vi "Zaxis_ZRaxis_Test.vi"() -> ()   [LabVIEW 2019]
uses:
  WSCbot_V3_Toolkit.lvlibp/WSCBOTV3_Toolkit/MotorControl/LowLevel/ZaxisSlideSet.vi
  WSCbot_V3_Toolkit.lvlibp/WSCBOTV3_Toolkit/MotorControl/LowLevel/ZRaxisRotatingSet.vi
  WSCbot_V3_Toolkit.lvlibp
panel:
  in  "TargetHight(deg)":dbl format="%#_13g"
  in  "TargetABSHight(mm)":dbl format="%#_13g"
  in  "error in (no error)":errorcluster
  in  "Stop Button":bool
  in  "上下測試":bool
  in  "旋轉測試":bool
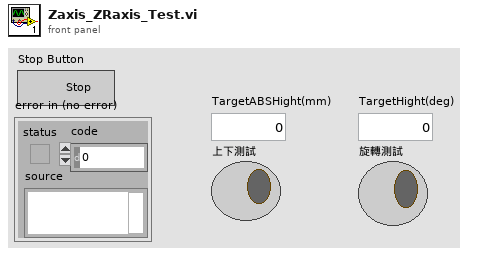
[diagram p1: front panel]
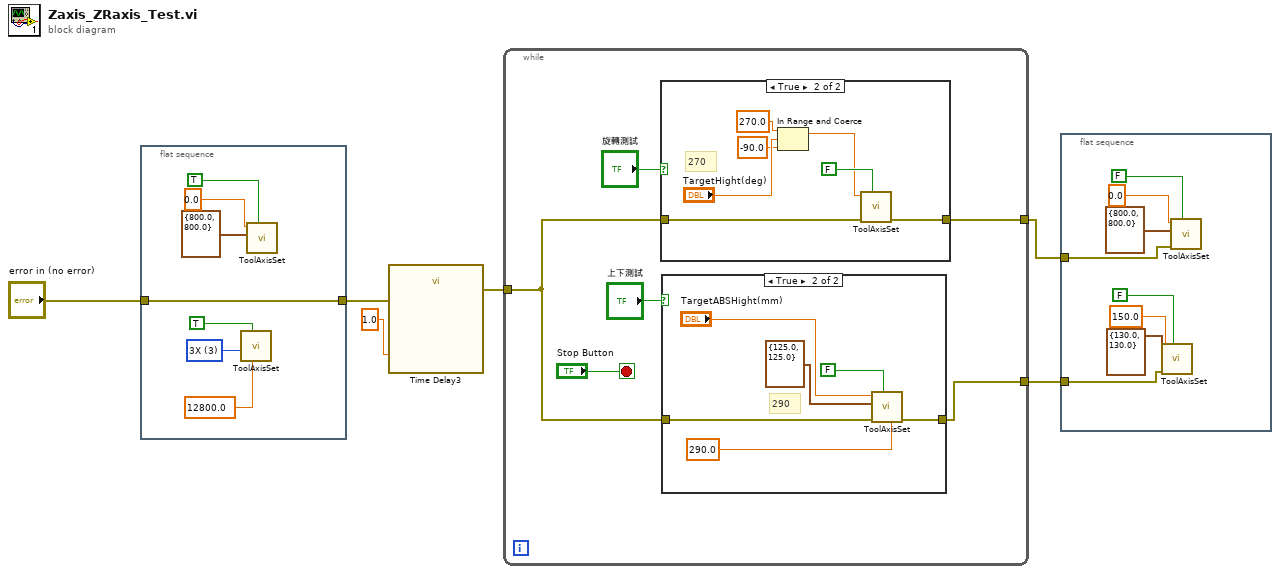
[diagram p0: block diagram]
diagram:
  n1 = flat-sequence {
    tunnel: [w7] -> w4
    tunnel: "error in (no error)" -> [w7]
    frame #0 {
      w11 = u16 3 items=["0X", "1X", "2X", "3X"] ("findHomeVel (times)")
      n2 = call-poly "ToolAxisSet.vi"("Pulse/rev"=12800.0, "Reset"=TRUE, "findHomeVel (times)"=w11) -> ()  [unwired: 7 in, 2 out]
      n3 = call-poly "ToolAxisSet.vi"("Reset"=TRUE, "Velocity(deg/s)&ACC(deg/ss)"=cluster{"Velocity(cm/s)":dbl, "ACC(cm/ss)":dbl} {"Velocity(cm/s)"=800.0, "ACC(cm/ss)"=800.0}, "TargetHight(deg)"=0.0) -> ()  [unwired: 7 in, 2 out]
    }
  }
  n4 = call "Time Delay3"("error in (no error)"=w4, "Delay Time (s)"=1.0) -> ("error out"=w3:errorcluster)  [unwired: 9 in]
  n5 = while {
    tunnel: w3 -> [w16]
    tunnel: [w15] -> w2
    tunnel: [w14] -> w1
    stop <- "Stop Button" stop-if-true
    n6 = case shown="True" "旋轉測試" {
      tunnel: w16 -> [w27 w34]
      tunnel: [w27 w33] -> w15
      frame False {
      }
      frame True {
        # "270"
        n7 = In Range and Coerce(upper limit=270.0, x="TargetHight(deg)", lower limit=-90.0) -> (coerced(x)=w28:dbl)  [unwired: 1 out]
        n8 = call-poly "ToolAxisSet.vi"("Reset"=FALSE, "error in"=w34, "TargetHight(deg)"=w28) -> ("error out"=w33:errorcluster)  [unwired: 7 in, 1 out]
      }
    }
    n9 = case shown="True" "上下測試" {
      tunnel: w16 -> [w20 w23]
      tunnel: [w20 w22] -> w14
      frame False {
      }
      frame True {
        # "290"
        n10 = call-poly "ToolAxisSet.vi"("upper limit"=290.0, "Reset"=FALSE, "error in"=w23, "Velocity(mm/s)&ACC(mm/ss)"=cluster{"Velocity(cm/s)":dbl, "ACC(cm/ss)":dbl} {"Velocity(cm/s)"=125.0, "ACC(cm/ss)"=125.0}, "TargetABSHight(mm)"="TargetABSHight(mm)") -> ("error out"=w22:errorcluster)  [unwired: 5 in, 1 out]
      }
    }
  }
  n11 = flat-sequence {
    tunnel: w2 -> [w36]
    tunnel: w1 -> [w35]
    frame #0 {
      n12 = call-poly "ToolAxisSet.vi"("Reset"=FALSE, "error in"=w35, "Velocity(mm/s)&ACC(mm/ss)"=cluster{"Velocity(cm/s)":dbl, "ACC(cm/ss)":dbl} {"Velocity(cm/s)"=130.0, "ACC(cm/ss)"=130.0}, "TargetABSHight(mm)"=150.0) -> ()  [unwired: 6 in, 2 out]
      n13 = call-poly "ToolAxisSet.vi"("Reset"=FALSE, "error in"=w36, "Velocity(deg/s)&ACC(deg/ss)"=cluster{"Velocity(cm/s)":dbl, "ACC(cm/ss)":dbl} {"Velocity(cm/s)"=800.0, "ACC(cm/ss)"=800.0}, "TargetHight(deg)"=0.0) -> ()  [unwired: 6 in, 2 out]
    }
  }
